vi "DSP_CreateWindowFunction.vi"(0 "Board Handle":u64, 5 "Window Type":u32(ring) items=["FFT_WINDOW_NONE", "FFT_WINDOW_HANNING", "FFT_WINDOW_HAMMING", "FFT_WINDOW_BLACKMAN", "FFT_WINDOW_BLACKMAN_HARRIS", "FFT_WINDOW_BARTLETT"], 7 "Samples Per Record":u32, 9 "Max Samples Per Record":u32, 11 "error in (no error)":errorcluster) -> (4 "Board Handle Out":u64, 6 "values out":u16[](array[numeric]), 15 "error out":errorcluster)   [LabVIEW 2018]
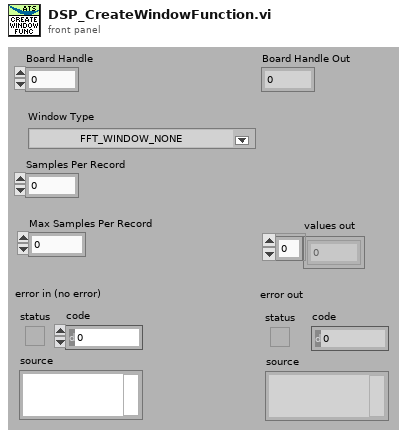
[diagram p1: front panel]
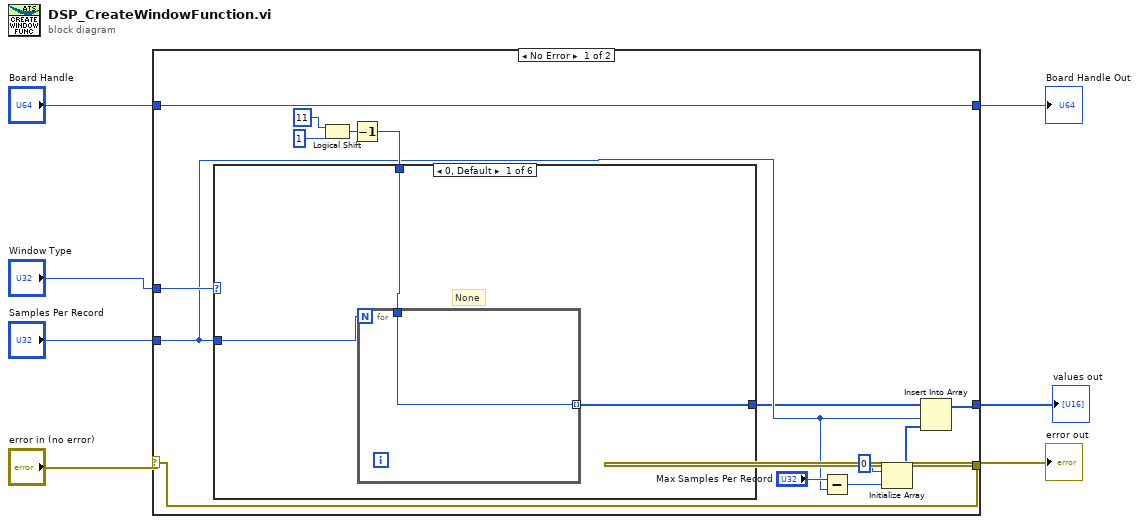
[diagram p0: block diagram]
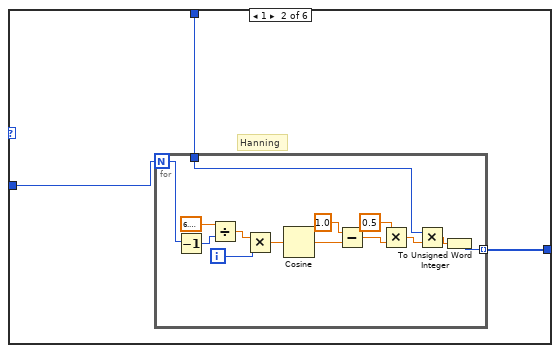
[diagram p2: hidden frame]
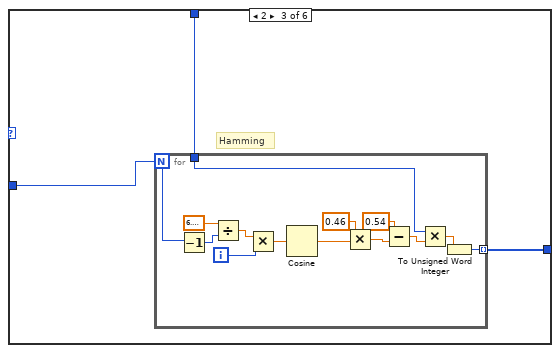
[diagram p3: hidden frame]
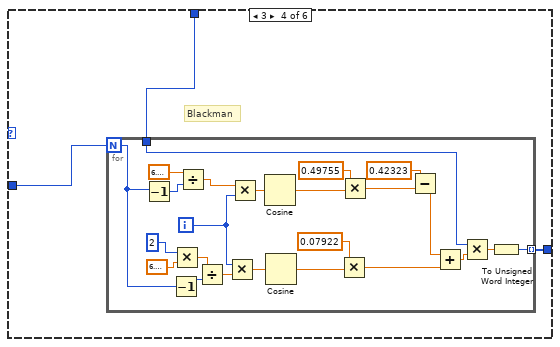
[diagram p4: hidden frame]
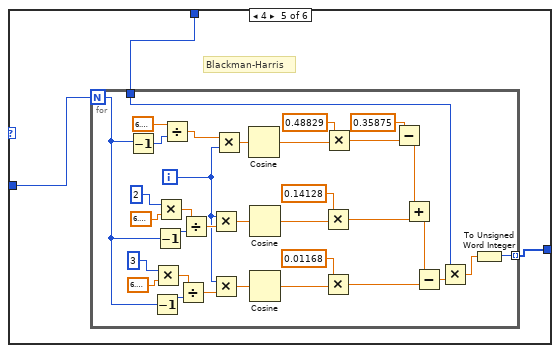
[diagram p5: hidden frame]
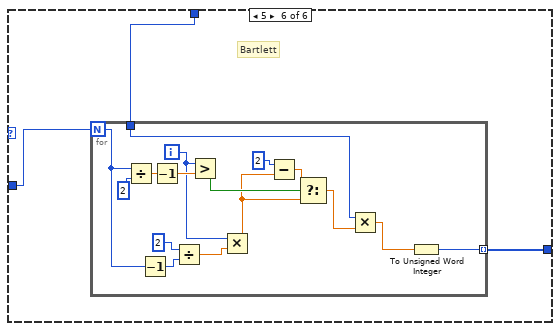
[diagram p6: hidden frame]
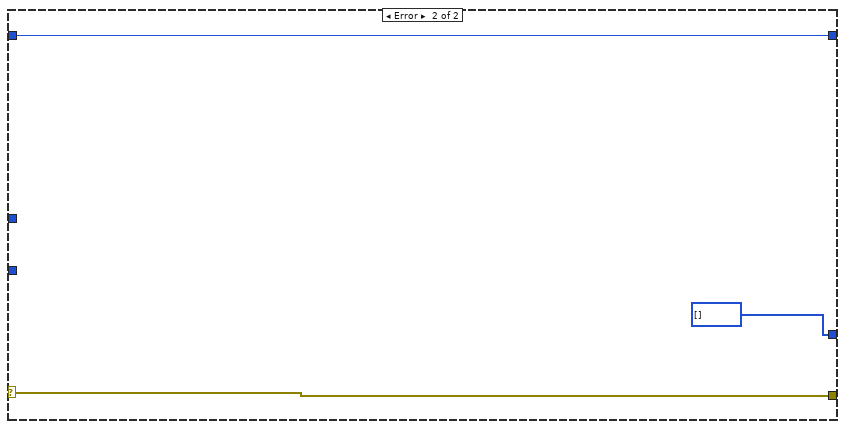
[diagram p7: hidden frame]
diagram:
  n1 = case shown="No Error" "error in (no error)" {
    selector: "error in (no error)" -> [w15 w145]
    tunnel: [w15 w145] -> w6
    tunnel: [w21 w144] -> w5
    tunnel: "Board Handle" -> [w21 w144]
    tunnel: "Samples Per Record" -> [w13 _]
    tunnel: "Window Type" -> [w17 _]
    tunnel: [w11 u16[] []] -> w1
    frame No Error {
      n2 = Logical Shift(y=11, x=u32 1) -> (x << y=w18:u32)
      n3 = Decrement(x=w18) -> (x-1=w16:u32)
      n4 = case shown="0, Default" w17 {
        tunnel: w13 -> [w24 w27 w44 w61 w88 w126]
        tunnel: [w23 w26 w43 w60 w87 w124] -> w12
        tunnel: w16 -> [w22 w28 w45 w62 w89 w125]
        frame 0, Default {
          # "None"
          n5 = for {
            N: w24 -> [_]
            tunnel: [w25] -> w23 mode=indexing
            tunnel: w22 -> [w25]
          }
        }
        frame 1 {
          # "Hanning"
          n6 = for {
            N: w27 -> [w40]
            tunnel: w28 -> [w31]
            tunnel: [w29] -> w26 mode=indexing
            i -> [w38]
            n7 = Decrement(x=w40) -> (x-1=w41:i32)
            n8 = Divide(x=6.283185307179586, y=w41) -> (x/y=w39:dbl)
            n9 = Multiply(x=w39, y=w38) -> (x*y=w37:dbl)
            n10 = Cosine(x=w37) -> (cos(x)=w36:dbl)
            n11 = Subtract(x=1.0, y=w36) -> (x-y=w33:dbl)
            n12 = Multiply(x=0.5, y=w33) -> (x*y=w32:dbl)
            n13 = Multiply(x=w31, y=w32) -> (x*y=w30:dbl)
            n14 = To Unsigned Word Integer(number=w30) -> (unsigned 16bit integer=w29:u16)
          }
        }
        frame 2 {
          # "Hamming"
          n15 = for {
            N: w44 -> [w57]
            tunnel: w45 -> [w51]
            tunnel: [w46] -> w43 mode=indexing
            i -> [w55]
            n16 = Decrement(x=w57) -> (x-1=w58:i32)
            n17 = Divide(x=6.283185307179586, y=w58) -> (x/y=w56:dbl)
            n18 = Multiply(x=w56, y=w55) -> (x*y=w54:dbl)
            n19 = Cosine(x=w54) -> (cos(x)=w48:dbl)
            n20 = Multiply(x=0.46, y=w48) -> (x*y=w50:dbl)
            n21 = Subtract(x=0.54, y=w50) -> (x-y=w52:dbl)
            n22 = Multiply(x=w51, y=w52) -> (x*y=w47:dbl)
            n23 = To Unsigned Word Integer(number=w47) -> (unsigned 16bit integer=w46:u16)
          }
        }
        frame 3 {
          # "Blackman"
          n24 = for {
            N: w61 -> [w73]
            tunnel: w62 -> [w81]
            tunnel: [w64] -> w60 mode=indexing
            i -> [w70]
            n25 = Decrement(x=w73) -> (x-1=w85:i32)
            n26 = Decrement(x=w73) -> (x-1=w77:i32)
            n27 = Multiply(x=2, y=6.283185307179586) -> (x*y=w74:dbl)
            n28 = Divide(x=6.283185307179586, y=w85) -> (x/y=w84:dbl)
            n29 = Divide(x=w74, y=w77) -> (x/y=w71:dbl)
            n30 = Multiply(x=w70, y=w71) -> (x*y=w72:dbl)
            n31 = Multiply(x=w84, y=w70) -> (x*y=w83:dbl)
            n32 = Cosine(x=w83) -> (cos(x)=w78:dbl)
            n33 = Cosine(x=w72) -> (cos(x)=w68:dbl)
            n34 = Multiply(x=0.07922, y=w68) -> (x*y=w66:dbl)
            n35 = Multiply(x=0.49755, y=w78) -> (x*y=w80:dbl)
            n36 = Subtract(x=0.42323, y=w80) -> (x-y=w65:dbl)
            n37 = Add(x=w65, y=w66) -> (x+y=w67:dbl)
            n38 = Multiply(x=w81, y=w67) -> (x*y=w63:dbl)
            n39 = To Unsigned Word Integer(number=w63) -> (unsigned 16bit integer=w64:u16)
          }
        }
        frame 4 {
          # "Blackman-Harris"
          n40 = for {
            N: w88 -> [w100]
            tunnel: w89 -> [w118]
            tunnel: [w91] -> w87 mode=indexing
            i -> [w96]
            n41 = Decrement(x=w100) -> (x-1=w122:i32)
            n42 = Decrement(x=w100) -> (x-1=w104:i32)
            n43 = Multiply(x=3, y=6.283185307179586) -> (x*y=w101:dbl)
            n44 = Decrement(x=w100) -> (x-1=w114:i32)
            n45 = Multiply(x=2, y=6.283185307179586) -> (x*y=w111:dbl)
            n46 = Divide(x=6.283185307179586, y=w122) -> (x/y=w121:dbl)
            n47 = Divide(x=w101, y=w104) -> (x/y=w95:dbl)
            n48 = Divide(x=w111, y=w114) -> (x/y=w109:dbl)
            n49 = Multiply(x=w96, y=w109) -> (x*y=w110:dbl)
            n50 = Multiply(x=w96, y=w95) -> (x*y=w99:dbl)
            n51 = Multiply(x=w121, y=w96) -> (x*y=w120:dbl)
            n52 = Cosine(x=w120) -> (cos(x)=w115:dbl)
            n53 = Cosine(x=w110) -> (cos(x)=w107:dbl)
            n54 = Cosine(x=w99) -> (cos(x)=w97:dbl)
            n55 = Multiply(x=0.14128, y=w107) -> (x*y=w106:dbl)
            n56 = Multiply(x=0.01168, y=w97) -> (x*y=w92:dbl)
            n57 = Multiply(x=0.48829, y=w115) -> (x*y=w117:dbl)
            n58 = Subtract(x=0.35875, y=w117) -> (x-y=w105:dbl)
            n59 = Add(x=w105, y=w106) -> (x+y=w93:dbl)
            n60 = Subtract(x=w93, y=w92) -> (x-y=w94:dbl)
            n61 = Multiply(x=w118, y=w94) -> (x*y=w90:dbl)
            n62 = To Unsigned Word Integer(number=w90) -> (unsigned 16bit integer=w91:u16)
          }
        }
        frame 5 {
          # "Bartlett"
          n63 = for {
            N: w126 -> [w137]
            tunnel: w125 -> [w130]
            tunnel: [w127] -> w124 mode=indexing
            i -> [w136]
            n64 = Divide(x=w137, y=2) -> (x/y=w141:dbl)
            n65 = Decrement(x=w137) -> (x-1=w138:i32)
            n66 = Decrement(x=w141) -> (x-1=w140:dbl)
            n67 = Divide(x=2, y=w138) -> (x/y=w135:dbl)
            n68 = Greater?(x=w136, y=w140) -> (0:w139:bool)
            n69 = Multiply(x=w136, y=w135) -> (x*y=w131:dbl)
            n70 = Subtract(x=2, y=w131) -> (x-y=w132:dbl)
            n71 = Select(t=w132, s=w139, f=w131) -> (s? t:f=w129:dbl)
            n72 = Multiply(x=w130, y=w129) -> (x*y=w128:dbl)
            n73 = To Unsigned Word Integer(number=w128) -> (unsigned 16bit integer=w127:u16)
          }
        }
      }
      n74 = Subtract(x="Max Samples Per Record", y=w13) -> (x-y=w10:u32)
      n75 = Initialize Array(u16 0, w10) -> (w8:u16[])
      n76 = Insert Into Array(array=w12, index=w13, new element=w8) -> (w11:u32[])
    }
    frame Error {
    }
  }
  "Board Handle Out" <- w5
  "error out" <- w6
  "values out" <- w1
